vi "Read UID.vi"(11 "Transport in":refnum<class "Transport.lvclass">) -> (2 "UID":i32)   [LabVIEW 2020, in "jettl.lvlib" / "Transport.lvclass"]
uses:
  Transport.lvclass
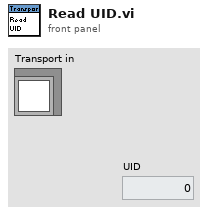
[diagram p1: front panel]
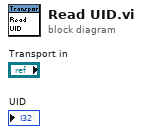
[diagram p0: block diagram]
diagram:
